vi "FindMassResolution.vi"   [LabVIEW 2012]
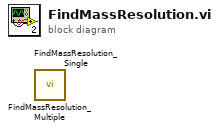
[diagram p0: block diagram]
diagram:
  n1 = call "FindMassResolution_Multiple.vi"() -> ()  [unwired: 10 in, 2 out]
  n2 = call "FindMassResolution_Single.vi"() -> ()  [unwired: 10 in, 2 out]
